vi "For.vi"() -> ()   [LabVIEW 2020]
panel:
  out "Valores":i32
  out "I":i32
  in  "Control de I":i32
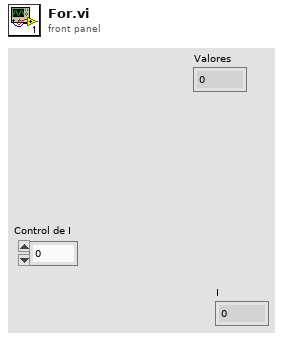
[diagram p1: front panel]
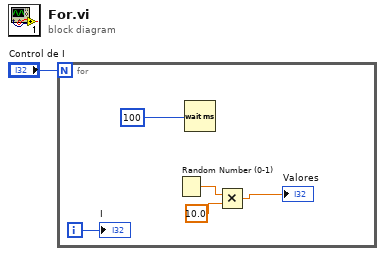
[diagram p0: block diagram]
diagram:
  n1 = for {
    N: "Control de I" -> [_]
    i -> [w6]
    n2 = Random Number (0-1)() -> (number: 0 to 1=w3:dbl)
    n3 = Wait (ms)(milliseconds to wait=100) -> ()  [unwired: 1 out]
    n4 = Multiply(x=w3, y=10.0) -> (x*y=→"Valores":dbl)
    "I" <- w6
  }
